vi "PM-P-Process_main.vi"(8 "error out":errorcluster, 11 "init_cluster":T1) -> (0 "error out out":errorcluster)   [LabVIEW 2018]
uses:
  init-close/PM-init-data_cluster.ctl
  init-close/PM-init-user_events.ctl
  init-close/PM-common-heartrate_data.ctl
  init-close/PM-common-peak-detect_settings.ctl
  PM-P-loop_data.ctl
  PM-P-user_events.ctl
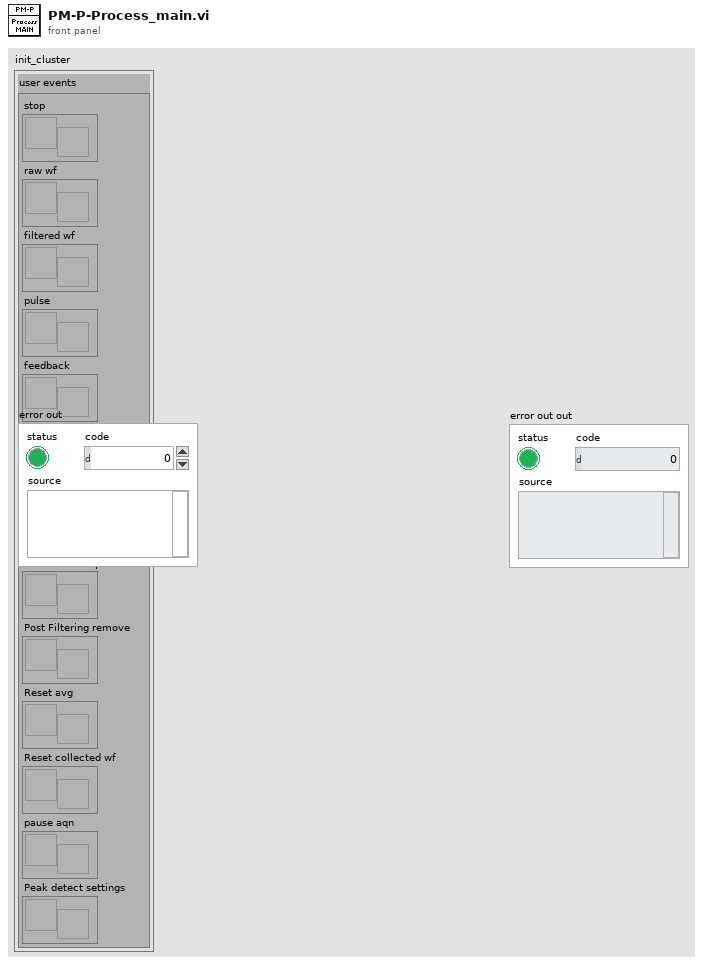
[diagram p1: front panel]
types:
  T1 = typedef "PM-init-data_cluster.ctl" = cluster{"user events":T2}
  T2 = typedef "PM-init-user_events.ctl" = cluster{"stop":refnum<user-event>, "raw wf":refnum<user-event>, "filtered wf":refnum<user-event>, "pulse":refnum<user-event>, "feedback":refnum<user-event>, "raw collected wf":refnum<user-event>, "avg sample size":refnum<user-event>, "Collected sample size":refnum<user-event>, "Post Filtering remove":refnum<user-event>, "Reset avg":refnum<user-event>, "Reset collected wf":refnum<user-event>, "pause aqn":refnum<user-event>, "Peak detect settings":refnum<user-event>}
  T3 = typedef "PM-P-user_events.ctl" = cluster{"Stop":refnum<user-event>, "raw collected wf":refnum<user-event>, "pulse":refnum<user-event>, "filtered wf":refnum<user-event>, "feedback":refnum<user-event>}
  T4 = typedef "PM-P-loop_data.ctl" = cluster{"user event":T3, "Raw waveform":waveform(dbl), "Sample size [s] (10)":i32, "Addition signal to remove (0) [s]":dbl, "Filtered waveform":waveform(dbl), "# samples to average (10)":i32, "heartrate [bpm]":dbl, "heartrate avg [bpm]":dbl, "heartrate avg array":dbl[], "Top":dbl, "Bottom":dbl, "Manual peak detect?":bool}
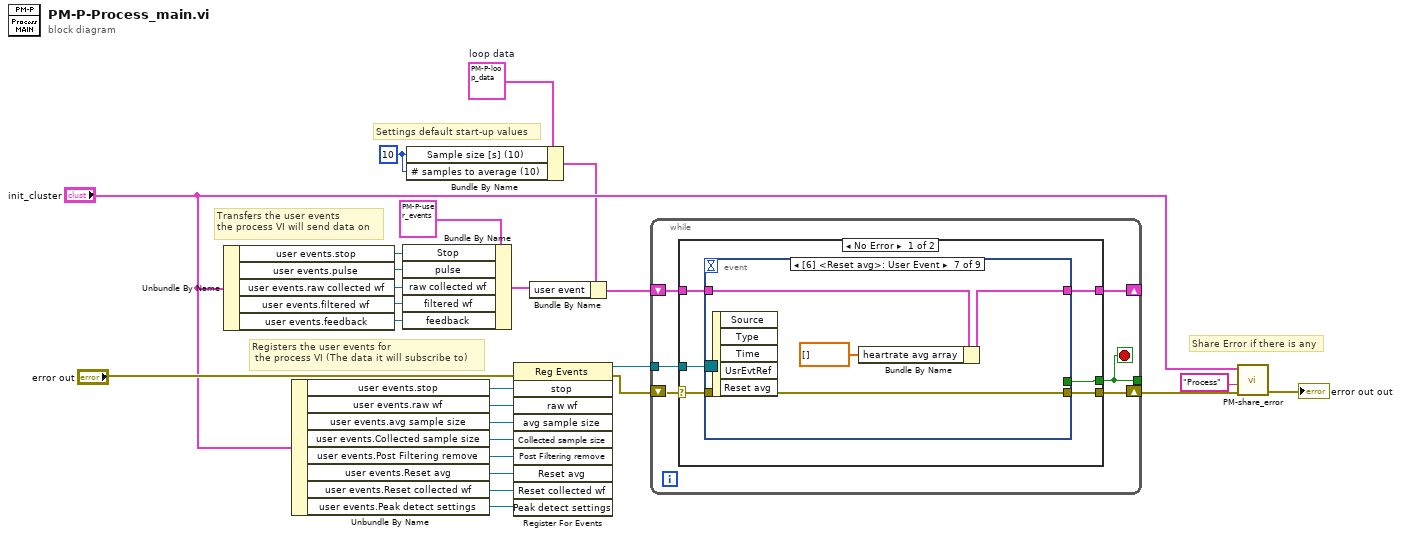
[diagram p0: block diagram]
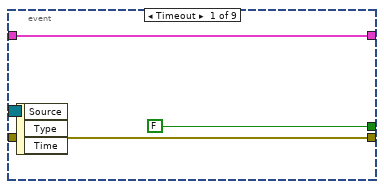
[diagram p2: hidden frame]
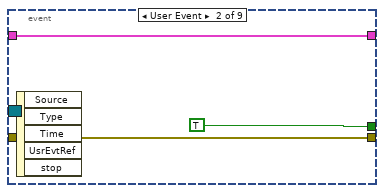
[diagram p3: hidden frame]
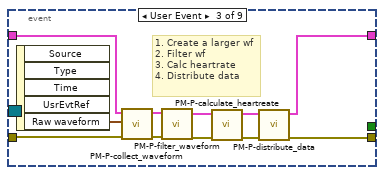
[diagram p4: hidden frame]
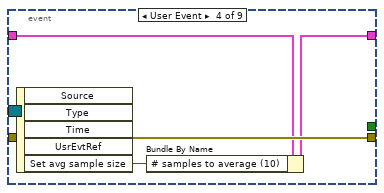
[diagram p5: hidden frame]
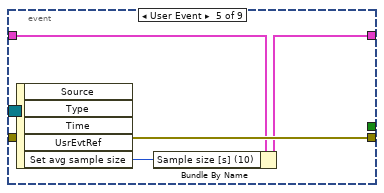
[diagram p6: hidden frame]
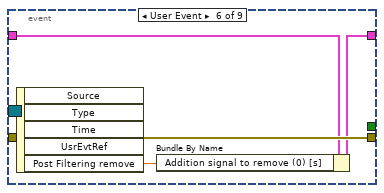
[diagram p7: hidden frame]
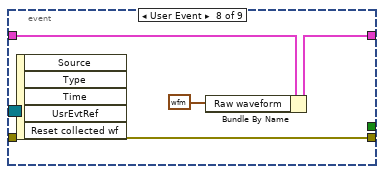
[diagram p8: hidden frame]
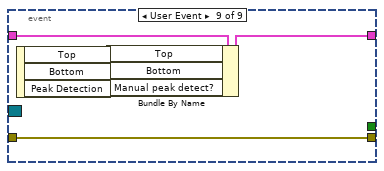
[diagram p9: hidden frame]
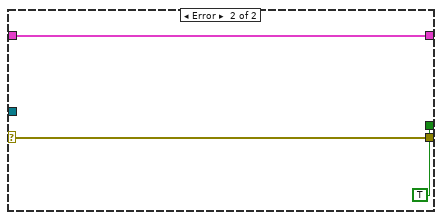
[diagram p10: hidden frame]
diagram:
  w2 = 10 ("Sample size [s] (10)")
  w12 = T4 {"user event"={"Stop"=refnum, "raw collected wf"=refnum, "pulse"=refnum, "filtered wf"=refnum, "feedback"=refnum}, "Raw waveform"={"t0"=timestamp(0 s since 1904-01-01), "dt"=1.0, "Y"=[]}, "Sample size [s] (10)"=0, "Addition signal to remove (0) [s]"=0.0, "Filtered waveform"={"t0"=timestamp(0 s since 1904-01-01), "dt"=1.0, "Y"=[]}, "# samples to average (10)"=0, "heartrate [bpm]"=0.0, "heartrate avg [bpm]"=0.0, "heartrate avg array"=[], "Top"=0.0, "Bottom"=0.0, "Manual peak detect?"=FALSE}  # loop data
  # "Share Error if there is any"
  # "Settings default start-up values"
  # "Registers the user events for\n the process VI (The data it will subscribe to)"
  # "Transfers the user events\nthe process VI will send data on"
  n1 = Unbundle By Name("init_cluster") -> ("user events.stop"=w21:refnum<user-event>, "user events.pulse"=w20:refnum<user-event>, "user events.raw collected wf"=w15:refnum<user-event>, "user events.filtered wf"=w14:refnum<user-event>, "user events.feedback"=w9:refnum<user-event>)
  n2 = Unbundle By Name("init_cluster") -> ("user events.stop"=w25:refnum<user-event>, "user events.raw wf"=w23:refnum<user-event>, "user events.avg sample size"=w8:refnum<user-event>, "user events.Collected sample size"=w7:refnum<user-event>, "user events.Post Filtering remove"=w6:refnum<user-event>, "user events.Reset avg"=w5:refnum<user-event>, "user events.Reset collected wf"=w4:refnum<user-event>, "user events.Peak detect settings"=w1:refnum<user-event>)
  n3 = Bundle By Name(cluster=T3 {"Stop"=refnum, "raw collected wf"=refnum, "pulse"=refnum, "filtered wf"=refnum, "feedback"=refnum} ("user event"), "Stop"=w21, "pulse"=w20, "raw collected wf"=w15, "filtered wf"=w14, "feedback"=w9) -> (w10:T3)
  n4 = Bundle By Name(cluster=w12, "Sample size [s] (10)"=w2, "# samples to average (10)"=w2) -> (w3:T4)
  n5 = register-events(error in="error out", w25, w23, w8, w7, w6, w5, w4, w1) -> (reference out=w24:refnum<event-registration>, error out=w26:errorcluster)  [unwired: 1 in]
  n6 = Bundle By Name(cluster=w3, "user event"=w10) -> (w11:T4)
  n7 = while {
    tunnel: [w31] -> _
    shift-right: [w30] -> w18
    shift-left: w26 -> [w32]
    tunnel: w24 -> [w29]
    shift-right: [w27] -> _
    shift-left: w11 -> [w28]
    stop <- w31 stop-if-true
    n8 = case shown="No Error" w32 {
      selector: w32 -> [w36 w83]
      tunnel: [w38 TRUE] -> w31
      tunnel: [w37 w83] -> w30
      tunnel: w29 -> [w35 _]
      tunnel: w28 -> [w34 w82]
      tunnel: [w33 w82] -> w27
      frame No Error {
        n9 = event shown="[6] <Reset avg>: User Event" {
          selector: w35 -> [_ _ _ _ _ _ _ _ _]
          dyn-events: _ -> [_ _ _ _ _ _ _ _ _]
          timeout: _ -> [_ _ _ _ _ _ _ _ _]
          tunnel: [FALSE TRUE _ _ _ _ _ _ _] -> w38
          tunnel: [w40 w44 w45 w59 w63 w67 w71 w75 w81] -> w37
          tunnel: w36 -> [w40 w44 w51 w59 w63 w67 w71 w75 w81]
          tunnel: w34 -> [w39 w42 w54 w58 w62 w66 w70 w74 w80]
          tunnel: [w39 w42 w46 w57 w61 w65 w69 w73 w79] -> w33
          event Timeout {
            n10 = event-data() -> ()  [unwired: 1 in, 3 out]
          }
          event User Event {
            n11 = event-data() -> ()  [unwired: 1 in, 5 out]
          }
          event User Event {
            # "1. Create a larger wf\n2. Filter wf\n3. Calc heartrate\n4. Distribute data"
            n12 = event-data() -> ("Raw waveform"=w55:waveform(dbl))  [unwired: 1 in, 4 out]
            n13 = call "PM-P-collect_waveform.vi"("error in (no error)"=w51, "New data in"=w55, "loop data in"=w54) -> ("error out"=w52:errorcluster, "loop data out"=w53:T4)  [unwired: 7 in]
            n14 = call "PM-P-filter_waveform.vi"("error in (no error)"=w52, "loop data"=w53) -> ("error out"=w50:errorcluster, "loop data"=w49:T4)  [unwired: 8 in]
            n15 = call "PM-P-calculate_heartreate.vi"("error in (no error)"=w50, "loop data"=w49) -> ("error out"=w47:errorcluster, "loop data out"=w48:T4)  [unwired: 8 in]
            n16 = call "PM-P-distribute_data.vi"("error in (no error)"=w47, "loop data"=w48) -> ("error out"=w45:errorcluster, "loop data"=w46:T4)  [unwired: 8 in]
          }
          event User Event {
            n17 = event-data() -> ("Set avg sample size"=w56:u32)  [unwired: 1 in, 4 out]
            n18 = Bundle By Name(cluster=w58, "# samples to average (10)"=w56) -> (w57:T4)
          }
          event User Event {
            n19 = event-data() -> ("Set avg sample size"=w60:u32)  [unwired: 1 in, 4 out]
            n20 = Bundle By Name(cluster=w62, "Sample size [s] (10)"=w60) -> (w61:T4)
          }
          event User Event {
            n21 = event-data() -> ("Post Filtering remove"=w64:dbl)  [unwired: 1 in, 4 out]
            n22 = Bundle By Name(cluster=w66, "Addition signal to remove (0) [s]"=w64) -> (w65:T4)
          }
          event User Event {
            n23 = event-data() -> ()  [unwired: 1 in, 5 out]
            n24 = Bundle By Name(cluster=w70, "heartrate avg array"=dbl[] []) -> (w69:T4)
          }
          event User Event {
            n25 = event-data() -> ()  [unwired: 1 in, 5 out]
            n26 = Bundle By Name(cluster=w74, "Raw waveform"=waveform(dbl) {"t0"=timestamp(0 s since 1904-01-01), "dt"=1.0, "Y"=[]}) -> (w73:T4)
          }
          event User Event {
            n27 = event-data() -> ("Top"=w78:dbl, "Bottom"=w77:dbl, "Peak Detection"=w76:bool)  [unwired: 1 in]
            n28 = Bundle By Name(cluster=w80, "Top"=w78, "Bottom"=w77, "Manual peak detect?"=w76) -> (w79:T4)
          }
        }
      }
      frame Error {
      }
    }
  }
  n29 = call "PM-share_error.vi"("error in (no error)"=w18, "module name"="Process", "init_cluster"="init_cluster") -> ("error out"=→"error out out":errorcluster)  [unwired: 8 in]
